vi "Switch all LEDs.vi"(8 "error in":errorcluster, 10 "Live channel":enum8{"Red", "Green", "Blue", "UV", ""}(ring)=enum."", 11 "LED handle in":refnum<visa-resource-name>) -> (0 "error out":errorcluster {"code" format="%.0x"}, 3 "LED handle out":refnum<visa-resource-name> caption="instrument handle out")   [LabVIEW 2017]
panel:
  in  "Switching delay (ms)":u32=200
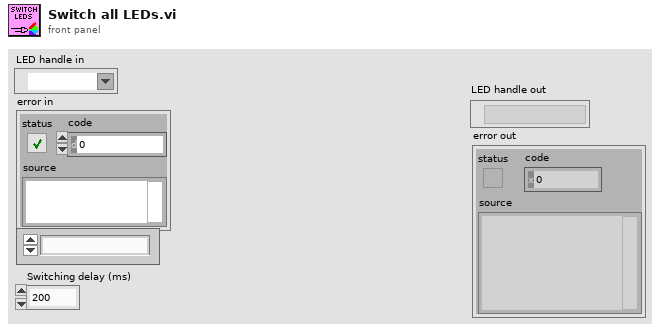
[diagram p1: front panel]
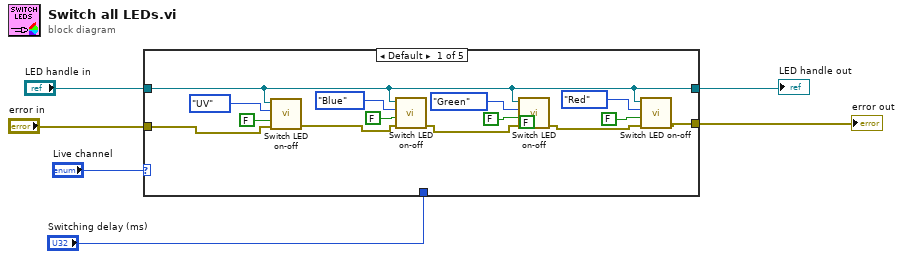
[diagram p0: block diagram]
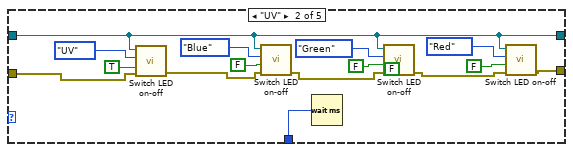
[diagram p2: hidden frame]
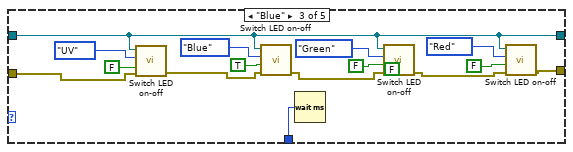
[diagram p3: hidden frame]
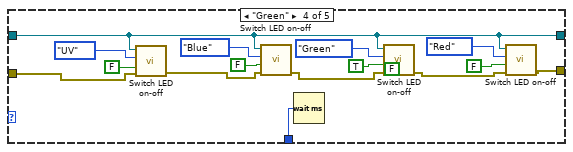
[diagram p4: hidden frame]
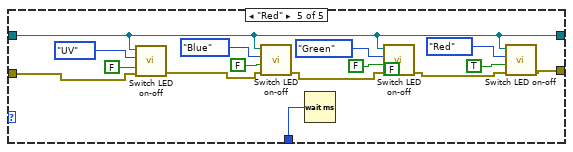
[diagram p5: hidden frame]
diagram:
  n1 = case shown="Default" "Live channel" {
    tunnel: [w10 w25 w40 w55 w70] -> w6
    tunnel: "LED handle in" -> [w10 w25 w40 w55 w70]
    tunnel: "error in" -> [w18 w33 w48 w63 w78]
    tunnel: [w11 w26 w41 w56 w71] -> w2
    tunnel: "Switching delay (ms)" -> [_ w21 w36 w51 w66]
    frame Default {
      (unwired) FALSE ("Laser On/Off")
      n2 = call "Switch LED on-off.vi"("error in"=w18, "LED On/Off"=FALSE ("Laser On/Off"), "LED"=enum8{"Red", "UV", "Green", "Blue"}."UV", "LED handle in"=w10) -> ("error out"=w14:errorcluster)  [unwired: 6 in, 1 out]
      n3 = call "Switch LED on-off.vi"("error in"=w14, "LED On/Off"=FALSE ("Laser On/Off"), "LED"=enum8{"Red", "UV", "Green", "Blue"}."Blue", "LED handle in"=w10) -> ("error out"=w13:errorcluster)  [unwired: 6 in, 1 out]
      n4 = call "Switch LED on-off.vi"("error in"=w13, "LED On/Off"=FALSE ("Laser On/Off"), "LED"=enum8{"Red", "UV", "Green", "Blue"}."Green", "LED handle in"=w10) -> ("error out"=w12:errorcluster)  [unwired: 6 in, 1 out]
      n5 = call "Switch LED on-off.vi"("error in"=w12, "LED On/Off"=FALSE ("Laser On/Off"), "LED"=enum8{"Red", "UV", "Green", "Blue"}."Red", "LED handle in"=w10) -> ("error out"=w11:errorcluster)  [unwired: 6 in, 1 out]
    }
    frame "UV" {
      (unwired) FALSE ("Laser On/Off")
      n6 = call "Switch LED on-off.vi"("error in"=w33, "LED On/Off"=TRUE ("Laser On/Off"), "LED"=enum8{"Red", "UV", "Green", "Blue"}."UV", "LED handle in"=w25) -> ("error out"=w29:errorcluster)  [unwired: 6 in, 1 out]
      n7 = call "Switch LED on-off.vi"("error in"=w29, "LED On/Off"=FALSE ("Laser On/Off"), "LED"=enum8{"Red", "UV", "Green", "Blue"}."Blue", "LED handle in"=w25) -> ("error out"=w28:errorcluster)  [unwired: 6 in, 1 out]
      n8 = Wait (ms)(milliseconds to wait=w21) -> ()  [unwired: 1 out]
      n9 = call "Switch LED on-off.vi"("error in"=w28, "LED On/Off"=FALSE ("Laser On/Off"), "LED"=enum8{"Red", "UV", "Green", "Blue"}."Green", "LED handle in"=w25) -> ("error out"=w27:errorcluster)  [unwired: 6 in, 1 out]
      n10 = call "Switch LED on-off.vi"("error in"=w27, "LED On/Off"=FALSE ("Laser On/Off"), "LED"=enum8{"Red", "UV", "Green", "Blue"}."Red", "LED handle in"=w25) -> ("error out"=w26:errorcluster)  [unwired: 6 in, 1 out]
    }
    frame "Blue" {
      (unwired) FALSE ("Laser On/Off")
      n11 = call "Switch LED on-off.vi"("error in"=w48, "LED On/Off"=FALSE ("Laser On/Off"), "LED"=enum8{"Red", "UV", "Green", "Blue"}."UV", "LED handle in"=w40) -> ("error out"=w44:errorcluster)  [unwired: 6 in, 1 out]
      n12 = call "Switch LED on-off.vi"("error in"=w44, "LED On/Off"=TRUE ("Laser On/Off"), "LED"=enum8{"Red", "UV", "Green", "Blue"}."Blue", "LED handle in"=w40) -> ("error out"=w43:errorcluster)  [unwired: 6 in, 1 out]
      n13 = Wait (ms)(milliseconds to wait=w36) -> ()  [unwired: 1 out]
      n14 = call "Switch LED on-off.vi"("error in"=w43, "LED On/Off"=FALSE ("Laser On/Off"), "LED"=enum8{"Red", "UV", "Green", "Blue"}."Green", "LED handle in"=w40) -> ("error out"=w42:errorcluster)  [unwired: 6 in, 1 out]
      n15 = call "Switch LED on-off.vi"("error in"=w42, "LED On/Off"=FALSE ("Laser On/Off"), "LED"=enum8{"Red", "UV", "Green", "Blue"}."Red", "LED handle in"=w40) -> ("error out"=w41:errorcluster)  [unwired: 6 in, 1 out]
    }
    frame "Green" {
      (unwired) FALSE ("Laser On/Off")
      n16 = call "Switch LED on-off.vi"("error in"=w63, "LED On/Off"=FALSE ("Laser On/Off"), "LED"=enum8{"Red", "UV", "Green", "Blue"}."UV", "LED handle in"=w55) -> ("error out"=w59:errorcluster)  [unwired: 6 in, 1 out]
      n17 = call "Switch LED on-off.vi"("error in"=w59, "LED On/Off"=FALSE ("Laser On/Off"), "LED"=enum8{"Red", "UV", "Green", "Blue"}."Blue", "LED handle in"=w55) -> ("error out"=w58:errorcluster)  [unwired: 6 in, 1 out]
      n18 = Wait (ms)(milliseconds to wait=w51) -> ()  [unwired: 1 out]
      n19 = call "Switch LED on-off.vi"("error in"=w58, "LED On/Off"=TRUE ("Laser On/Off"), "LED"=enum8{"Red", "UV", "Green", "Blue"}."Green", "LED handle in"=w55) -> ("error out"=w57:errorcluster)  [unwired: 6 in, 1 out]
      n20 = call "Switch LED on-off.vi"("error in"=w57, "LED On/Off"=FALSE ("Laser On/Off"), "LED"=enum8{"Red", "UV", "Green", "Blue"}."Red", "LED handle in"=w55) -> ("error out"=w56:errorcluster)  [unwired: 6 in, 1 out]
    }
    frame "Red" {
      (unwired) FALSE ("Laser On/Off")
      n21 = call "Switch LED on-off.vi"("error in"=w78, "LED On/Off"=FALSE ("Laser On/Off"), "LED"=enum8{"Red", "UV", "Green", "Blue"}."UV", "LED handle in"=w70) -> ("error out"=w74:errorcluster)  [unwired: 6 in, 1 out]
      n22 = call "Switch LED on-off.vi"("error in"=w74, "LED On/Off"=FALSE ("Laser On/Off"), "LED"=enum8{"Red", "UV", "Green", "Blue"}."Blue", "LED handle in"=w70) -> ("error out"=w73:errorcluster)  [unwired: 6 in, 1 out]
      n23 = Wait (ms)(milliseconds to wait=w66) -> ()  [unwired: 1 out]
      n24 = call "Switch LED on-off.vi"("error in"=w73, "LED On/Off"=FALSE ("Laser On/Off"), "LED"=enum8{"Red", "UV", "Green", "Blue"}."Green", "LED handle in"=w70) -> ("error out"=w72:errorcluster)  [unwired: 6 in, 1 out]
      n25 = call "Switch LED on-off.vi"("error in"=w72, "LED On/Off"=TRUE ("Laser On/Off"), "LED"=enum8{"Red", "UV", "Green", "Blue"}."Red", "LED handle in"=w70) -> ("error out"=w71:errorcluster)  [unwired: 6 in, 1 out]
    }
  }
  "LED handle out" <- w6
  "error out" <- w2
